vi "T 3 (SubVI).vi"(10 "arg":dbl format="%#_13g") -> (2 "matrix":dbl[][](array[numeric]))   [LabVIEW 2017]
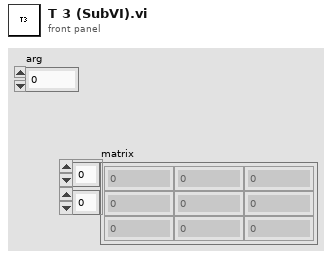
[diagram p1: front panel]
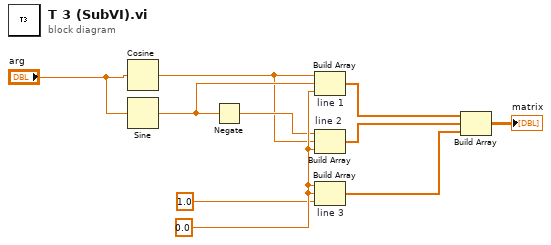
[diagram p0: block diagram]
diagram:
  w5 = 0.0 ("element")
  n1 = Cosine(x="arg") -> (cos(x)=w1:dbl)
  n2 = Sine(x="arg") -> (sin(x)=w4:dbl)
  n3 = Negate(x=w4) -> (-x=w2:dbl)
  n4 = Build Array "line 1"(w1, w4, w5) -> (w7:dbl[])
  n5 = Build Array "line 2"(w2, w1, w5) -> (w8:dbl[])
  n6 = Build Array "line 3"(w5, w5, 1.0 ("element")) -> (w9:dbl[])
  n7 = Build Array(w7, w8, w9) -> (→"matrix":dbl[][])
